vi "Start Event Loop.vi"(10 "Quit Event":refnum<user-event>) -> ()   [LabVIEW 2014, in "LQ Core.lvlib" / "LQCoreEngine.lvclass"]
uses:
  LQCoreEngine.lvclass
  Signal Packet_Void Bool.ctl
  Signal Packet_I32.ctl
  Signal Packet_String.ctl
  Signal Packet_DBL.ctl
  Connection Action.ctl
  Signal Data Type.ctl
  LQ Core.lvlib
panel:
  # "Copyright (c) 2016 Sze Howe Koh\n\nThis Source Code Form is subject to the terms of the Mozilla Public\nLicense, v. 2.0. If a copy of the MPL was not distributed with this\nfile, You can obtain one at http://mozilla.org/MPL/2.0/."
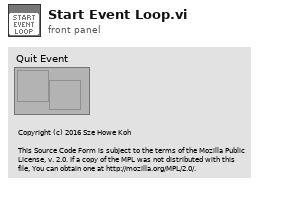
[diagram p1: front panel]
types:
  T1 = typedef "LQ Core.lvlib/LQCoreEngine.lvclass/Signal Packet_DBL.ctl" = cluster{"QObject Refnum":u64, "Signal Index":i64, "Signal Value":dbl}
  T2 = typedef "LQ Core.lvlib/LQCoreEngine.lvclass/Signal Packet_String.ctl" = cluster{"QObject Refnum":u64, "Signal Index":i64, "Signal Value":string}
  T3 = typedef "LQ Core.lvlib/LQCoreEngine.lvclass/Signal Packet_I32.ctl" = cluster{"QObject Refnum":u64, "Signal Index":i64, "Signal Value":i32}
  T4 = typedef "LQ Core.lvlib/LQCoreEngine.lvclass/Signal Packet_Void Bool.ctl" = cluster{"QObject Refnum":u64, "Signal Index":i64, "Signal Value":bool}
  T5 = typedef "LQ Core.lvlib/LQCoreEngine.lvclass/Signal Data Type.ctl" = enum16{"Void", "Bool", "I32", "DBL", "String"}
  T6 = typedef "LQ Core.lvlib/LQCoreEngine.lvclass/Connection Action.ctl" = enum16{"Init", "Add Connection", "Get Connections", "Clean Up"}
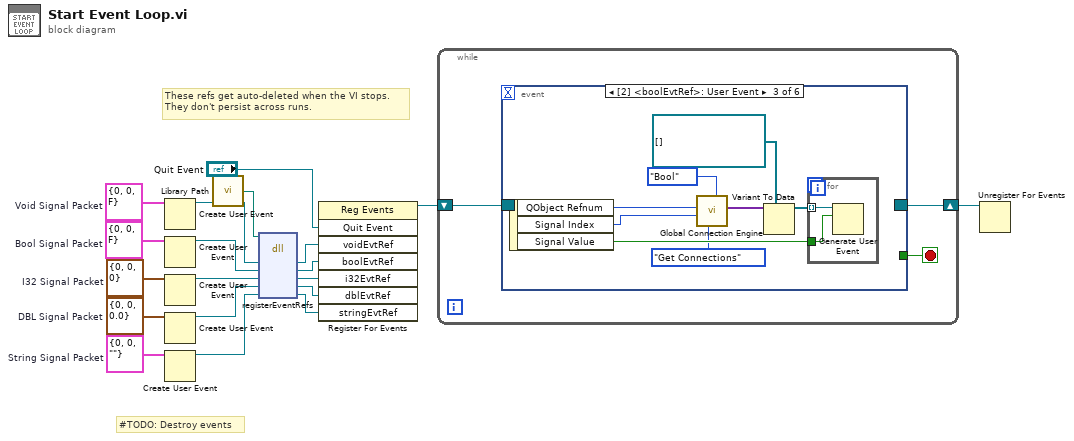
[diagram p0: block diagram]
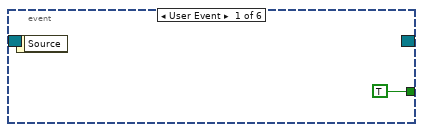
[diagram p2: hidden frame]
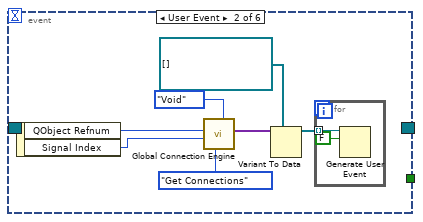
[diagram p3: hidden frame]
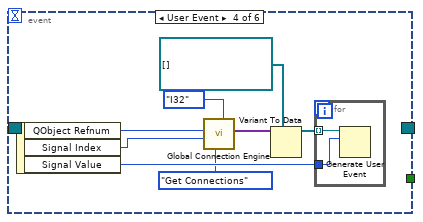
[diagram p4: hidden frame]
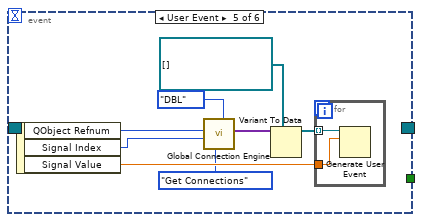
[diagram p5: hidden frame]
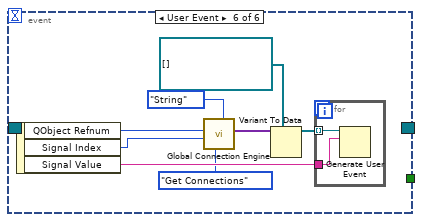
[diagram p6: hidden frame]
diagram:
  w3 = T1 {"QObject Refnum"=0, "Signal Index"=0, "Signal Value"=0.0}  # DBL Signal Packet
  w6 = T2 {"QObject Refnum"=0, "Signal Index"=0, "Signal Value"=""}  # String Signal Packet
  w7 = T3 {"QObject Refnum"=0, "Signal Index"=0, "Signal Value"=0}  # I32 Signal Packet
  w8 = T4 {"QObject Refnum"=0, "Signal Index"=0, "Signal Value"=FALSE}  # Bool Signal Packet
  w9 = T4 {"QObject Refnum"=0, "Signal Index"=0, "Signal Value"=FALSE}  # Void Signal Packet
  # "These refs get auto-deleted when the VI stops.\nThey don't persist across runs."
  # "#TODO: Destroy events"
  n1 = Create User Event(user event datatype=w9) -> (user event=w19:refnum<user-event>)  [unwired: 1 in, 1 out]
  n2 = Create User Event(user event datatype=w8) -> (user event=w18:refnum<user-event>)  [unwired: 1 in, 1 out]
  n3 = Create User Event(user event datatype=w7) -> (user event=w17:refnum<user-event>)  [unwired: 1 in, 1 out]
  n4 = Create User Event(user event datatype=w3) -> (user event=w2:refnum<user-event>)  [unwired: 1 in, 1 out]
  n5 = Create User Event(user event datatype=w6) -> (user event=w16:refnum<user-event>)  [unwired: 1 in, 1 out]
  n6 = call "Library Path.vi"() -> ("Library Path"=w4:path)
  n7 = dll-call lib="?" fn="registerEventRefs"(path in=w4, "voidEvtRef"=w19, "boolEvtRef"=w18, "i32EvtRef"=w17, "dblEvtRef"=w2, "stringEvtRef"=w16) -> ("voidEvtRef"=w15:refnum<user-event>, "boolEvtRef"=w14:refnum<user-event>, "i32EvtRef"=w13:refnum<user-event>, "dblEvtRef"=w1:refnum<user-event>, "stringEvtRef"=w12:refnum<user-event>)  [unwired: 3 in, 2 out]
  n8 = register-events("Quit Event", w15, w14, w13, w1, w12) -> (reference out=w11:refnum<event-registration>)  [unwired: 2 in, 1 out]
  n9 = while {
    shift-right: [w21] -> w10
    shift-left: w11 -> [w22]
    stop <- w20 stop-if-true
    n10 = event shown="[2] <boolEvtRef>: User Event" {
      selector: w22 -> [_ _ _ _ _ _]
      dyn-events: [_ _ _ _ _ _] -> w21
      timeout: _ -> [_ _ _ _ _ _]
      tunnel: [TRUE _ _ _ _ _] -> w20
      event User Event {
        n11 = event-data() -> ()  [unwired: 1 in, 1 out]
      }
      event User Event {
        n12 = event-data() -> ("QObject Refnum"=w27:u64, "Signal Index"=w26:i64)  [unwired: 1 in]
        n13 = call "Global Connection Engine.vi"("Receiver Data Type"=Signal_Data_Type."Void", "Connection Action"=Connection_Action."Get Connections", "Signal Index"=w26, "LQObject Manifestation"=w27) -> ("Receiver Channels Out"=w30:variant[])  [unwired: 7 in]
        n14 = Variant To Data(type=refnum<user-event>[] [], Variant=w30) -> (data=w28:refnum<user-event>[])  [unwired: 1 in, 1 out]
        n15 = for {
          tunnel: w28 -> [w32] mode=indexing
          n16 = Generate User Event(user event=w32, event data cluster=FALSE ("event data")) -> ()  [unwired: 2 in, 2 out]
        }
      }
      event User Event {
        n17 = event-data() -> ("QObject Refnum"=w36:u64, "Signal Index"=w35:i64, "Signal Value"=w37:bool)  [unwired: 1 in]
        n18 = call "Global Connection Engine.vi"("Receiver Data Type"=Signal_Data_Type."Bool", "Connection Action"=Connection_Action."Get Connections", "Signal Index"=w35, "LQObject Manifestation"=w36) -> ("Receiver Channels Out"=w40:variant[])  [unwired: 7 in]
        n19 = Variant To Data(type=refnum<user-event>[] [], Variant=w40) -> (data=w38:refnum<user-event>[])  [unwired: 1 in, 1 out]
        n20 = for {
          tunnel: w38 -> [w42] mode=indexing
          tunnel: w37 -> [w41]
          n21 = Generate User Event(user event=w42, event data cluster=w41) -> ()  [unwired: 2 in, 2 out]
        }
      }
      event User Event {
        n22 = event-data() -> ("QObject Refnum"=w45:u64, "Signal Index"=w46:i64, "Signal Value"=w47:i32)  [unwired: 1 in]
        n23 = call "Global Connection Engine.vi"("Receiver Data Type"=Signal_Data_Type."I32", "Connection Action"=Connection_Action."Get Connections", "Signal Index"=w46, "LQObject Manifestation"=w45) -> ("Receiver Channels Out"=w50:variant[])  [unwired: 7 in]
        n24 = Variant To Data(type=refnum<user-event>[] [], Variant=w50) -> (data=w48:refnum<user-event>[])  [unwired: 1 in, 1 out]
        n25 = for {
          tunnel: w48 -> [w52] mode=indexing
          tunnel: w47 -> [w51]
          n26 = Generate User Event(user event=w52, event data cluster=w51) -> ()  [unwired: 2 in, 2 out]
        }
      }
      event User Event {
        n27 = event-data() -> ("QObject Refnum"=w55:u64, "Signal Index"=w56:i64, "Signal Value"=w57:dbl)  [unwired: 1 in]
        n28 = call "Global Connection Engine.vi"("Receiver Data Type"=Signal_Data_Type."DBL", "Connection Action"=Connection_Action."Get Connections", "Signal Index"=w56, "LQObject Manifestation"=w55) -> ("Receiver Channels Out"=w60:variant[])  [unwired: 7 in]
        n29 = Variant To Data(type=refnum<user-event>[] [], Variant=w60) -> (data=w58:refnum<user-event>[])  [unwired: 1 in, 1 out]
        n30 = for {
          tunnel: w58 -> [w62] mode=indexing
          tunnel: w57 -> [w61]
          n31 = Generate User Event(user event=w62, event data cluster=w61) -> ()  [unwired: 2 in, 2 out]
        }
      }
      event User Event {
        n32 = event-data() -> ("QObject Refnum"=w65:u64, "Signal Index"=w66:i64, "Signal Value"=w67:string)  [unwired: 1 in]
        n33 = call "Global Connection Engine.vi"("Receiver Data Type"=Signal_Data_Type."String", "Connection Action"=Connection_Action."Get Connections", "Signal Index"=w66, "LQObject Manifestation"=w65) -> ("Receiver Channels Out"=w70:variant[])  [unwired: 7 in]
        n34 = Variant To Data(type=refnum<user-event>[] [], Variant=w70) -> (data=w68:refnum<user-event>[])  [unwired: 1 in, 1 out]
        n35 = for {
          tunnel: w68 -> [w72] mode=indexing
          tunnel: w67 -> [w71]
          n36 = Generate User Event(user event=w72, event data cluster=w71) -> ()  [unwired: 2 in, 2 out]
        }
      }
    }
  }
  n37 = Unregister For Events(event registration refnum=w10) -> ()  [unwired: 1 in, 1 out]
